vi "Receive Control Mouse Wheel.vi"(8 "error in (no error)":errorcluster, 10 "Control Mouse Wheel Msg":refnum<class "Control MouseWheelMsg.lvclass">, 11 "GarphView In":refnum<class "GarphView.lvclass">) -> (0 "error out":errorcluster, 3 "GarphView Out":refnum<class "GarphView.lvclass">)   [LabVIEW 2020, in "GarphView.lvlib" / "GarphView.lvclass"]
doc: "<License>\nCopyright © 2017 Composed Systems, LLC | All rights reserved\nwww.composed.io\n\nAuthor: Ethan Stern <ethan.stern@composed.io>\n\nThis software is provided \"AS IS\" WITHOUT WARRANTIES, either express or implied, AND IS FOR EDUCATIONAL PURPOSES ONLY.\n</License>"
uses:
  GarphView.lvclass
  C:/Program Files (x86)/National Instruments/LabVIEW 2020/vi.lib/ActorFramework/Actor/Actor.lvclass
  <vilib>/gpm_packages/@cs/mva-viewable/Source/ActorEvents/IEventAggregator Messages/Receive Control Mouse Wheel Msg/Control MouseWheelMsg.lvclass
  <vilib>/ActorFramework/Actor/Actor.lvclass/Actor.ctl
  <vilib>/ActorFramework/Message Enqueuer/Message Enqueuer.lvclass/Message Enqueuer.ctl
  GarphView.lvclass/GarphView.ctl
  <vilib>/gpm_packages/@cs/mva-viewable/Source/ActorEvents/IEventAggregator Messages/Receive Control Mouse Wheel Msg/Control MouseWheelMsg.lvclass/Control MouseWheelMsg.ctl
  <vilib>/ActorFramework/Message Enqueuer/Enqueue.vi
  <vilib>/ActorFramework/Message Enqueuer/Init from Existing Queue.vi
  GarphView Messages/Redraw Points and Path Msg/Redraw Points and Path Msg.lvclass
  C:/Program Files (x86)/National Instruments/LabVIEW 2020/vi.lib/ActorFramework/Message/Message.lvclass
  <vilib>/ActorFramework/Message Priority Queue/Priority Enqueue.vi
  <vilib>/ActorFramework/Message Enqueuer/Message Enqueuer.lvclass
  <vilib>/ActorFramework/Actor/Actor.lvclass
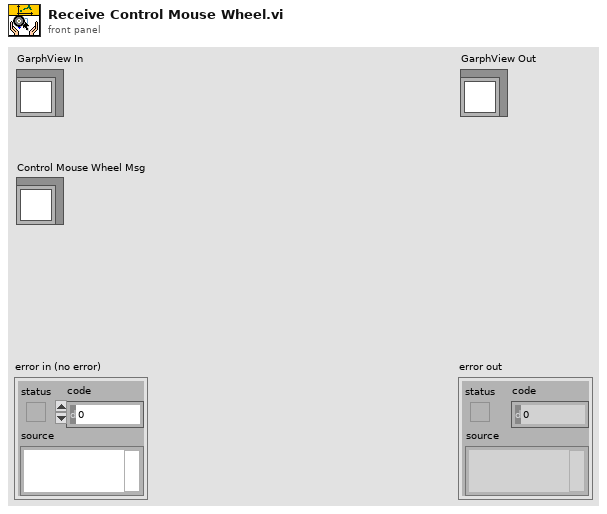
[diagram p1: front panel]
types:
  T1 = cluster{"Shift":bool, "Ctrl":bool, "Alt":bool, "Cmd":bool, "Opt":bool}
  T2 = typedef "LVRectTypeDef.ctl" = cluster{"Left":i16, "Top":i16, "Right":i16, "Bottom":i16}
  T3 = typedef "LVPoint32TypeDef.ctl" = cluster{"Horizontal":i32, "Vertical":i32}
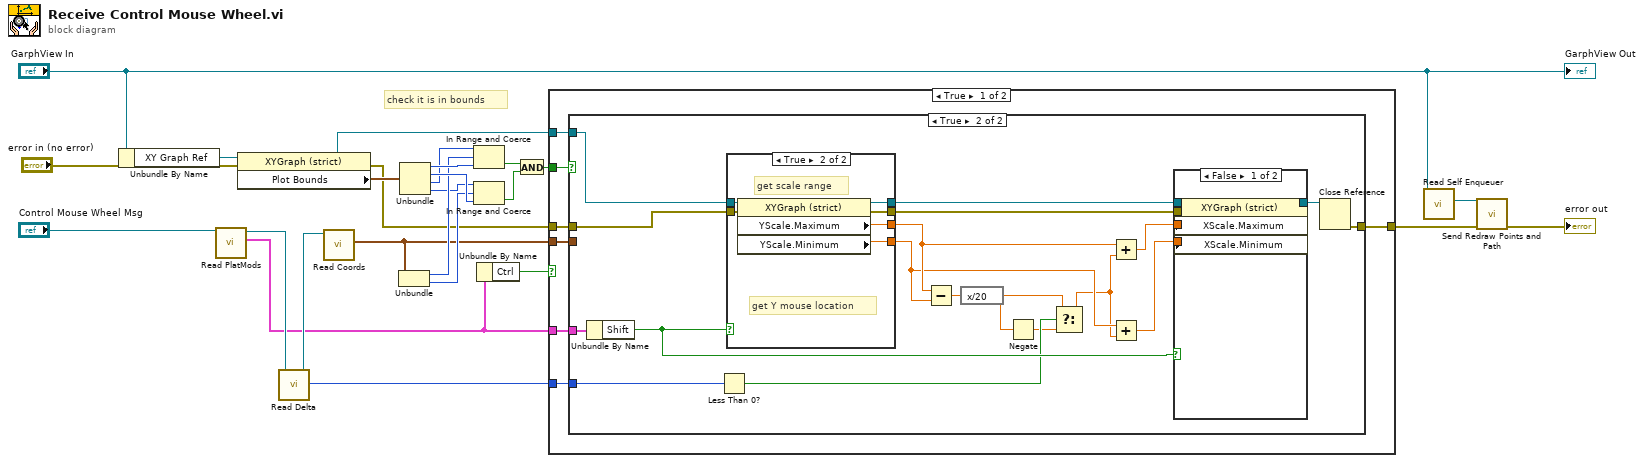
[diagram p0: block diagram]
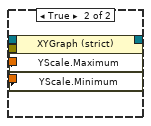
[diagram p3: hidden frame]
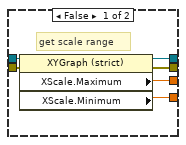
[diagram p4: hidden frame]
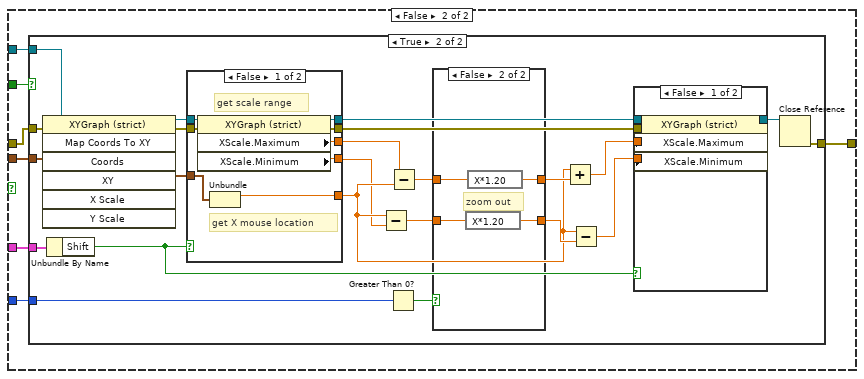
[diagram p5: hidden frame]
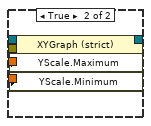
[diagram p7: hidden frame]
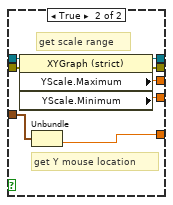
[diagram p8: hidden frame]
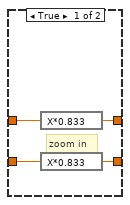
[diagram p9: hidden frame]
diagram:
  # "check it is in bounds"
  n1 = Unbundle By Name("GarphView In") -> ("XY Graph Ref"=w7:refnum<vi>)
  n2 = call <vilib>:"Read PlatMods.vi"("Control Mouse Wheel Msg in"="Control Mouse Wheel Msg") -> ("PlatMods"=w9:T1, "Control Mouse Wheel Msg out"=w13:refnum<class "Control MouseWheelMsg.lvclass">)  [unwired: 9 in]
  n3 = property on="Property Node" class="XYGraph (strict)"(reference=w7, error in="error in (no error)") -> (reference out=w15:refnum<vi>, error out=w6:errorcluster, "Plot Bounds"=w17:T2)
  n4 = call <vilib>:"Read Delta.vi"("Control Mouse Wheel Msg in"=w13) -> ("Delta"=w8:i32, "Control Mouse Wheel Msg out"=w12:refnum<class "Control MouseWheelMsg.lvclass">)  [unwired: 9 in]
  n5 = call <vilib>:"Read Coords.vi"("Control Mouse Wheel Msg in"=w12) -> ("Point32"=w10:T3)  [unwired: 9 in, 1 out]
  n6 = Unbundle(w10) -> ("Horizontal"=w22:i32, "Vertical"=w23:i32)
  n7 = Unbundle(w17) -> ("Left"=w25:i16, "Top"=w24:i16, "Right"=w21:i16, "Bottom"=w20:i16)
  n8 = In Range and Coerce(upper limit=w21, x=w22, lower limit=w25) -> (In Range?=w19:bool)  [unwired: 1 out]
  n9 = In Range and Coerce(upper limit=w20, x=w23, lower limit=w24) -> (In Range?=w18:bool)  [unwired: 1 out]
  n10 = Unbundle By Name(w9) -> ("Ctrl"=w14:bool)
  n11 = And(x=w19, y=w18) -> (x .and. y?=w16:bool)
  n12 = case shown="True" w14 {
    tunnel: w8 -> [w32 w80]
    tunnel: w6 -> [w31 w79]
    tunnel: w10 -> [w30 w78]
    tunnel: w16 -> [w29 w77]
    tunnel: w15 -> [w28 w76]
    tunnel: w9 -> [w27 w75]
    tunnel: [w26 w74] -> w2
    frame True {
      # "Holding CTRL - PAN Left and Right"
      n13 = case shown="True" w29 {
        tunnel: w32 -> [_ w47]
        tunnel: w28 -> [_ w43]
        tunnel: w31 -> [w33 w42]
        tunnel: w30 -> [_ _]
        tunnel: w27 -> [_ w45]
        tunnel: [w33 w34] -> w26
        frame False {
          # "not in the plot range, so ignore the scroll wheel"
        }
        frame True {
          n14 = Unbundle By Name(w45) -> ("Shift"=w44:bool)
          n15 = Less Than 0?(x=w47) -> (x < 0?=w38:bool)
          n16 = case shown="True" w44 {
            tunnel: [w67 w73] -> w40
            tunnel: [w66 w72] -> w39
            tunnel: [w65 w71] -> w49
            tunnel: [w64 w70] -> w48
            tunnel: w42 -> [w63 w69]
            tunnel: w43 -> [w62 w68]
            frame False {
              # "get scale range"
              n17 = property on="Property Node" class="XYGraph (strict)"(reference=w62, error in=w63) -> (reference out=w64:refnum<vi>, error out=w65:errorcluster, "XScale.Maximum"=w67:dbl, "XScale.Minimum"=w66:dbl)
            }
            frame True {
              # "get scale range"
              # "get Y mouse location"
              n18 = property on="Property Node" class="XYGraph (strict)"(reference=w68, error in=w69) -> (reference out=w70:refnum<vi>, error out=w71:errorcluster, "YScale.Maximum"=w73:dbl, "YScale.Minimum"=w72:dbl)
            }
          }
          n19 = Subtract(x=w40, y=w39) -> (x-y=w41:dbl)
          n20 = expression code="x/20"(w41) -> (w35:dbl)
          n21 = Negate(x=w35) -> (-x=w37:dbl)
          n22 = Select(t=w35, s=w38, f=w37) -> (s? t:f=w36:dbl)
          n23 = Add(x=w40, y=w36) -> (x+y=w50:dbl)
          n24 = Add(x=w39, y=w36) -> (x+y=w51:dbl)
          n25 = case shown="False" w44 {
            tunnel: w51 -> [w52 w61]
            tunnel: w50 -> [w53 w60]
            tunnel: w49 -> [w55 w59]
            tunnel: w48 -> [w56 w58]
            tunnel: [w54 w57] -> w46
            frame False {
              n26 = property on="Property Node" class="XYGraph (strict)"(reference=w56, error in=w55, "XScale.Maximum"=w53, "XScale.Minimum"=w52) -> (reference out=w54:refnum<vi>)  [unwired: 1 out]
            }
            frame True {
              n27 = property on="Property Node" class="XYGraph (strict)"(reference=w58, error in=w59, "YScale.Maximum"=w60, "YScale.Minimum"=w61) -> (reference out=w57:refnum<vi>)  [unwired: 1 out]
            }
          }
          n28 = Close Reference(reference=w46) -> (error out=w34:errorcluster)  [unwired: 1 in]
        }
      }
    }
    frame False {
      n29 = case shown="True" w77 {
        tunnel: w80 -> [_ w100]
        tunnel: w76 -> [_ w94]
        tunnel: w79 -> [w81 w93]
        tunnel: w78 -> [_ w92]
        tunnel: w75 -> [_ w91]
        tunnel: [w81 w82] -> w74
        frame False {
          # "not in the plot range, so ignore the scroll wheel"
        }
        frame True {
          n30 = invoke on="Invoke Node" class="XYGraph (strict)" method="Map Coords To XY"(reference=w94, error in=w93, "Coords"=w92) -> (reference out=w96:refnum<vi>, error out=w97:errorcluster, "XY"=w98:cluster{"X":dbl, "Y":dbl})  [unwired: 4 in, 4 out]
          n31 = Unbundle By Name(w91) -> ("Shift"=w90:bool)
          n32 = case shown="False" w90 {
            tunnel: [w122 w130] -> w87
            tunnel: [w121 w129] -> w84
            tunnel: [w120 w123] -> w85
            tunnel: [w119 w128] -> w102
            tunnel: [w118 w127] -> w101
            tunnel: w98 -> [w117 w126]
            tunnel: w97 -> [w116 w125]
            tunnel: w96 -> [w115 w124]
            frame False {
              # "get scale range"
              # "get X mouse location"
              n33 = property on="Property Node" class="XYGraph (strict)"(reference=w115, error in=w116) -> (reference out=w118:refnum<vi>, error out=w119:errorcluster, "XScale.Maximum"=w122:dbl, "XScale.Minimum"=w121:dbl)
              n34 = Unbundle(w117) -> ("X"=w120:dbl)  [unwired: 1 out]
            }
            frame True {
              # "get scale range"
              # "get Y mouse location"
              n35 = property on="Property Node" class="XYGraph (strict)"(reference=w124, error in=w125) -> (reference out=w127:refnum<vi>, error out=w128:errorcluster, "YScale.Maximum"=w130:dbl, "YScale.Minimum"=w129:dbl)
              n36 = Unbundle(w126) -> ("Y"=w123:dbl)  [unwired: 1 out]
            }
          }
          n37 = Subtract(x=w85, y=w84) -> (x-y=w83:dbl)
          n38 = Greater Than 0?(x=w100) -> (x > 0?=w99:bool)
          n39 = Subtract(x=w87, y=w85) -> (x-y=w86:dbl)
          n40 = case shown="False" w99 {
            tunnel: w86 -> [w134 w138]
            tunnel: [w133 w137] -> w103
            tunnel: w83 -> [w132 w136]
            tunnel: [w131 w135] -> w89
            frame True {
              # "zoom in"
              n41 = expression code="X*0.833"(w134) -> (w133:dbl)
              n42 = expression code="X*0.833"(w132) -> (w131:dbl)
            }
            frame False {
              # "zoom out"
              n43 = expression code="X*1.20"(w136) -> (w135:dbl)
              n44 = expression code="X*1.20"(w138) -> (w137:dbl)
            }
          }
          n45 = Add(x=w85, y=w103) -> (x+y=w104:dbl)
          n46 = Subtract(x=w85, y=w89) -> (x-y=w88:dbl)
          n47 = case shown="False" w90 {
            tunnel: w88 -> [w105 w114]
            tunnel: w104 -> [w106 w113]
            tunnel: w102 -> [w108 w112]
            tunnel: w101 -> [w109 w111]
            tunnel: [w107 w110] -> w95
            frame False {
              n48 = property on="Property Node" class="XYGraph (strict)"(reference=w109, error in=w108, "XScale.Maximum"=w106, "XScale.Minimum"=w105) -> (reference out=w107:refnum<vi>)  [unwired: 1 out]
            }
            frame True {
              n49 = property on="Property Node" class="XYGraph (strict)"(reference=w111, error in=w112, "YScale.Maximum"=w113, "YScale.Minimum"=w114) -> (reference out=w110:refnum<vi>)  [unwired: 1 out]
            }
          }
          n50 = Close Reference(reference=w95) -> (error out=w82:errorcluster)  [unwired: 1 in]
        }
      }
    }
  }
  n51 = call <vilib>:"Read Self Enqueuer.vi"("Actor"="GarphView In") -> ("Self Enqueuer"=w3:refnum<class "Message Enqueuer.lvclass">)  [unwired: 10 in]
  n52 = call "Send Redraw Points and Path.vi"("error in (no error)"=w2, "Message Enqueuer"=w3) -> ("error out"=→"error out":errorcluster)  [unwired: 8 in, 1 out]
  "GarphView Out" <- "GarphView In"
